vi "Sort Scan Parameters.vi"(8 "error in (no error)":errorcluster, 11 "SweepControl":refnum<class "SMO.SweepControl.lvclass">) -> (0 "error out":errorcluster, 1 "Sorted scan parameters":cluster{T5}[](array[cluster])=[{[{"Start"=0.14, "End"=-0.060000000000000005, "Step"=-0.060000000000000005, "Rate"=0.0, "Waveform type"=enum."linear", "wait (ms or K)"=10000.0, "Address"="Dev2/ao0", "channel"=1}]}, {[{"Start"=0.14, "End"=-0.060000000000000005, "Step"=-0.060000000000000005, "Rate"=0.0, "Waveform type"=enum."linear", "wait (ms or K)"=10000.0, "Address"="Dev2/ao0", "channel"=1}]}, {[{"Start"=0.14, "End"=-0.060000000000000005, "Step"=-0.060000000000000005, "Rate"=0.0, "Waveform type"=enum."linear", "wait (ms or K)"=10000.0, "Address"="Dev2/ao0", "channel"=1}, {"Start"=0.14, "End"=-0.060000000000000005, "Step"=-0.060000000000000005, "Rate"=0.0, "Waveform type"=enum."linear", "wait (ms or K)"=10000.0, "Address"="Dev2/ao0", "channel"=1}]}] {"?"."Rate" format="%.2f"; "?"."Step" format="%#_6p"; "?"."End" format="%#_6p"; "?"."Start" format="%#_6p"}, 2 "Sorted scan control":cluster{T7}[](array[cluster])=[{[{"Priority"=enum."Priority 0", "Scan name"=enum."Delay"}]}, {[{"Priority"=enum."Priority 1", "Scan name"=enum."Lockin Amplitude"}]}, {[{"Priority"=enum."Priority 2", "Scan name"=enum."Lockin Bias"}, {"Priority"=enum."Priority 2", "Scan name"=enum."Magnet Field"}]}], 3 "SweepControl":refnum<class "SMO.SweepControl.lvclass">)   [LabVIEW 2019, in "SMO.SweepControl.lvclass"]
uses:
  SMO.SweepControl.lvclass
  Typedefs/Cluster - ScanParamters.ctl
  Typedefs/ScanParamters.ctl
  Typedefs/Enum - Priority.ctl
  Typedefs/Enum - Action.ctl
  Typedefs/Cluster - ScanControl.ctl
  Typedefs/ScanControl.ctl
  Typedefs/Enum - PostAction - 2.ctl
  Typedefs/Cluster - Sweep Control.ctl
panel:
  out "Sorted scan parameters 2":cluster{"Scan parameters 2":T1[]}[](array[cluster]) {"Scan parameters 2"."Rate" format="%.2f"; "Scan parameters 2"."Step" format="%#_6p"; "Scan parameters 2"."End" format="%#_6p"; "Scan parameters 2"."Start" format="%#_6p"}
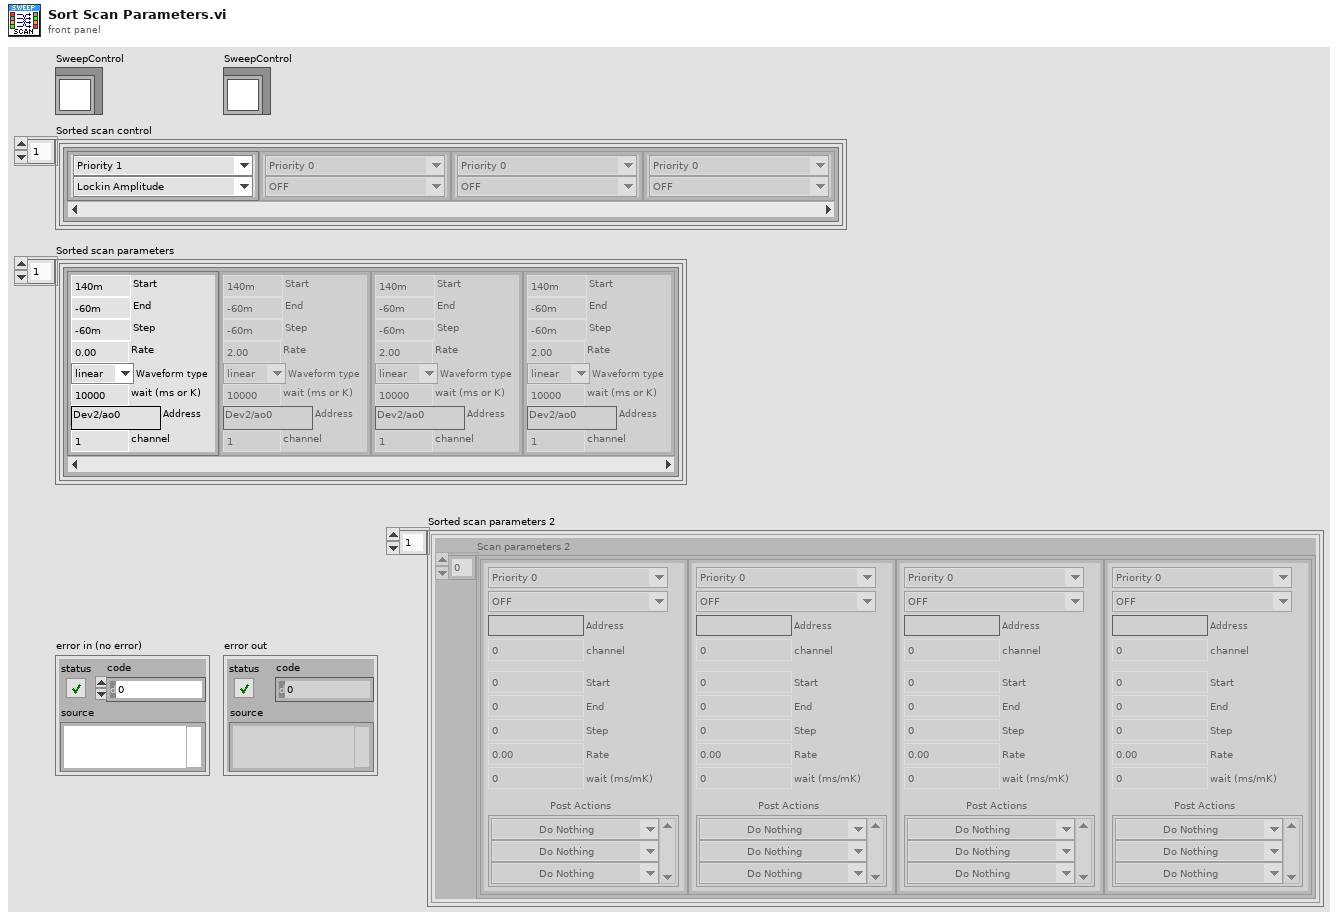
[diagram p1: front panel]
types:
  T1 = typedef "SMO.SweepControl.lvclass/Cluster - Sweep Control.ctl" = cluster{"Start":dbl, "End":dbl, "Step":dbl, "Rate":dbl, "wait (ms/mK)":u32, "Address":string, "Priority":T2, "Scan name":T3, "Post Actions":T4[], "channel":i32}
  T2 = typedef "SMO.SweepControl.lvclass/Enum - Priority.ctl" = enum16{"Priority 0", "Priority 1", "Priority 2", "Priority 3", "Priority 4", "Priority 5"}
  T3 = typedef "SMO.SweepControl.lvclass/Enum - Action.ctl" = enum16{"OFF", "time", "Lockin Amplitude", "Lockin Frequency", "Lockin Bias", "Delay", "Strain", "DAQ Bias", "Magnet Field", "Temperature", "MW f1", "MW f2", "MW Amplitude1", "MW Amplitude2"}
  T4 = typedef "SMO.SweepControl.lvclass/Enum - PostAction - 2.ctl" = enum16{"Do Nothing", "Wait (time)", "Wait (Temperature)", "Wait (<T ; B sweep)", "Wait (Magnet)"}
  T5 = typedef "SMO.SweepControl.lvclass/ScanParamters.ctl" = T6[]
  T6 = typedef "SMO.SweepControl.lvclass/Cluster - ScanParamters.ctl" = cluster{"Start":dbl, "End":dbl, "Step":dbl, "Rate":dbl, "Waveform type":enum16{"linear", "triangle", "power"}, "wait (ms or K)":dbl, "Address":string, "channel":i32}
  T7 = typedef "SMO.SweepControl.lvclass/ScanControl.ctl" = T8[]
  T8 = typedef "SMO.SweepControl.lvclass/Cluster - ScanControl.ctl" = cluster{"Priority":T2, "Scan name":T3}
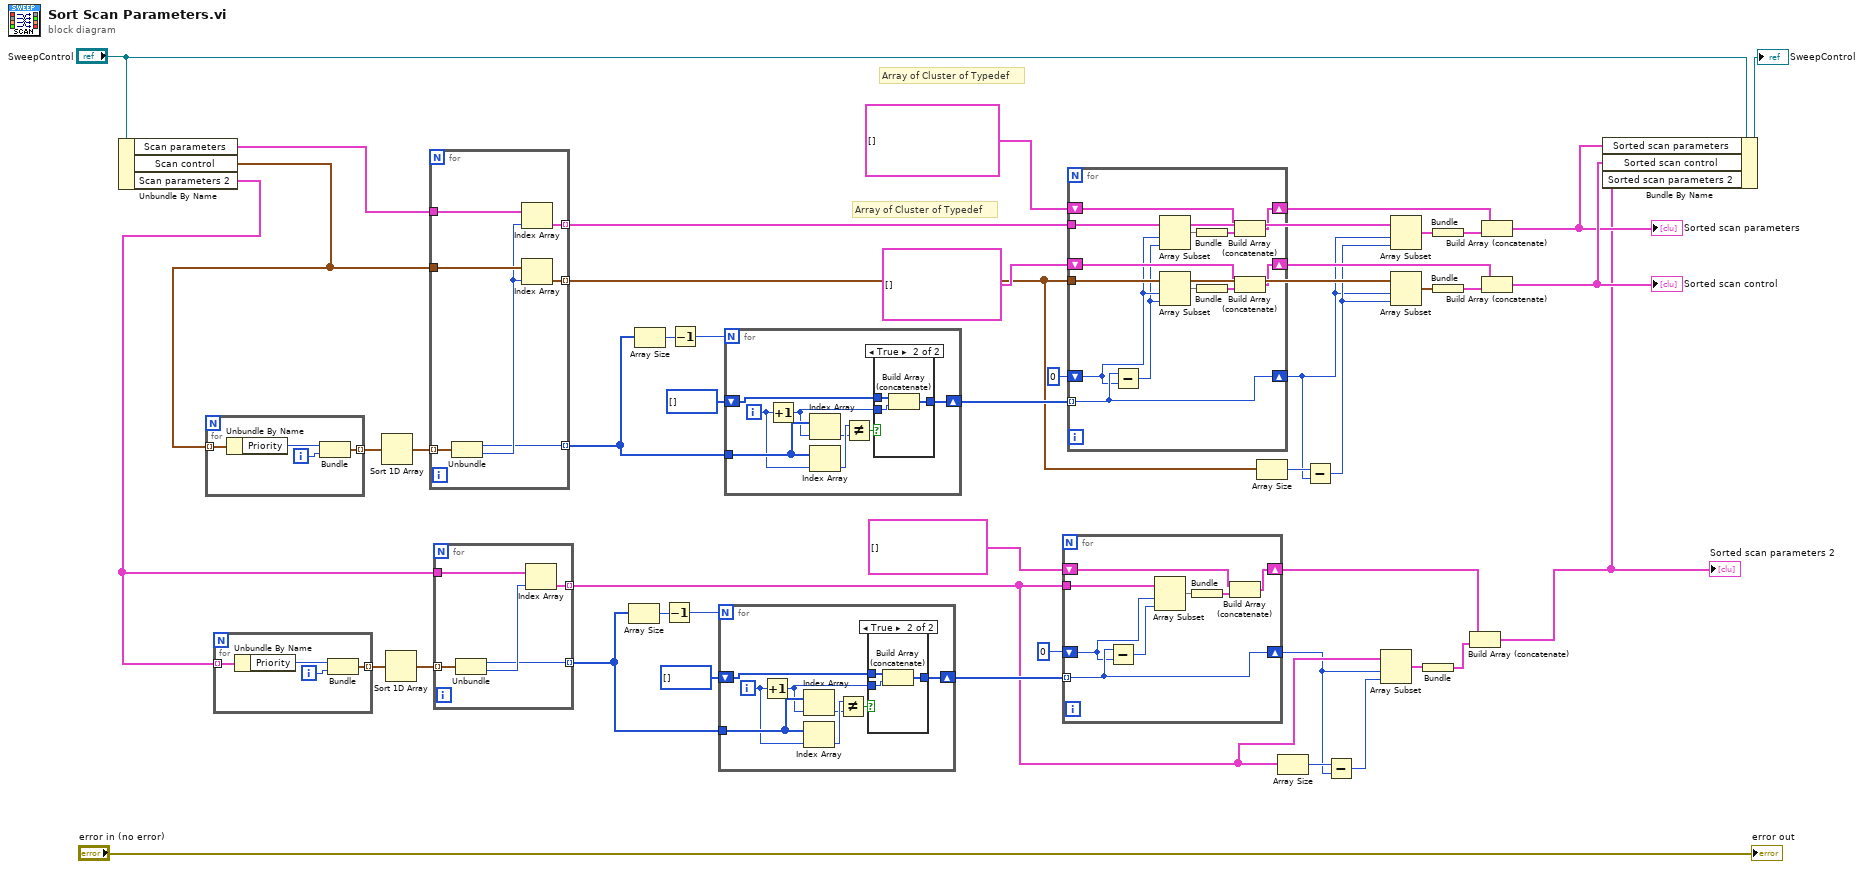
[diagram p0: block diagram]
diagram:
  # "Array of Cluster of Typedef"
  # "Array of Cluster of Typedef"
  n1 = Unbundle By Name("SweepControl") -> ("Scan parameters"=w25:T5, "Scan control"=w20:T7, "Scan parameters 2"=w18:T1[])
  n2 = for {
    tunnel: w20 -> [w47] mode=indexing
    tunnel: [w50] -> w46 mode=indexing
    i -> [w48]
    n3 = Unbundle By Name(w47) -> ("Priority"=w49:T2)
    n4 = Bundle("Priority"=w49, w48) -> (w50:cluster{"Priority":T2, i32})  [unwired: 1 in]
  }
  n5 = for {
    tunnel: w18 -> [w51] mode=indexing
    tunnel: [w54] -> w17 mode=indexing
    i -> [w52]
    n6 = Unbundle By Name(w51) -> ("Priority"=w53:T2)
    n7 = Bundle("Priority"=w53, w52) -> (w54:cluster{"Priority":T2, i32})  [unwired: 1 in]
  }
  n8 = Sort 1D Array(array=w46) -> (sorted array=w45:cluster{"Priority":T2, i32}[])
  n9 = Sort 1D Array(array=w17) -> (sorted array=w16:cluster{"Priority":T2, i32}[])
  n10 = for {
    tunnel: w45 -> [w61] mode=indexing
    tunnel: w20 -> [w60]
    tunnel: [w59] -> w35 mode=indexing
    tunnel: w25 -> [w58]
    tunnel: [w57] -> w31 mode=indexing
    tunnel: [w55] -> w42 mode=indexing
    n11 = Unbundle(w61) -> ("Priority"=w55:T2, w56:i32)
    n12 = Index Array(array=w58, index=w56) -> (element=w57:T6)
    n13 = Index Array(array=w60, index=w56) -> (element=w59:T8)
  }
  n14 = for {
    tunnel: w16 -> [w66] mode=indexing
    tunnel: w18 -> [w65]
    tunnel: [w64] -> w7 mode=indexing
    tunnel: [w62] -> w12 mode=indexing
    n15 = Unbundle(w66) -> ("Priority"=w62:T2, w63:i32)
    n16 = Index Array(array=w65, index=w63) -> (element=w64:T1)
  }
  n17 = Array Size(array=w12) -> (size(s)=w13:i32)
  n18 = Array Size(array=w42) -> (size(s)=w44:i32)
  n19 = Decrement(x=w13) -> (x-1=w14:i32)
  n20 = Decrement(x=w44) -> (x-1=w43:i32)
  n21 = for {
    N: w14 -> [_]
    tunnel: w12 -> [w74]
    shift-right: [w70] -> w10
    shift-left: i32[] [] -> [w69]
    i -> [w67]
    n22 = Increment(x=w67) -> (x+1=w68:i32)
    n23 = Index Array(array=w74, index=w68) -> (element=w71:T2)
    n24 = Index Array(array=w74, index=w67) -> (element=w73:T2)
    n25 = Not Equal?(x=w73, y=w71) -> (x != y?=w72:bool)
    n26 = case shown="True" w72 {
      tunnel: [w75 w78] -> w70
      tunnel: w69 -> [w75 w77]
      tunnel: w68 -> [_ w76]
      frame False {
      }
      frame True {
        n27 = Build Array (concatenate)(w77, w76) -> (w78:i32[])
      }
    }
  }
  n28 = for {
    N: w43 -> [_]
    tunnel: w42 -> [w86]
    shift-right: [w82] -> w39
    shift-left: i32[] [] -> [w81]
    i -> [w79]
    n29 = Increment(x=w79) -> (x+1=w80:i32)
    n30 = Index Array(array=w86, index=w80) -> (element=w83:T2)
    n31 = Index Array(array=w86, index=w79) -> (element=w85:T2)
    n32 = Not Equal?(x=w85, y=w83) -> (x != y?=w84:bool)
    n33 = case shown="True" w84 {
      tunnel: [w87 w90] -> w82
      tunnel: w81 -> [w87 w89]
      tunnel: w80 -> [_ w88]
      frame False {
      }
      frame True {
        n34 = Build Array (concatenate)(w89, w88) -> (w90:i32[])
      }
    }
  }
  n35 = for {
    tunnel: w10 -> [w98] mode=indexing
    shift-right: [w98] -> w3
    shift-left: 0 -> [w96]
    tunnel: w7 -> [w97]
    shift-right: [w93] -> w4
    shift-left: cluster{"Scan parameters 2":T1[]}[] [] -> [w92]
    n36 = Subtract(x=w98, y=w96) -> (x-y=w95:i32)
    n37 = Array Subset(array=w97, index=w96, length=w95) -> (w94:T1[])
    n38 = Bundle(w94) -> (w91:cluster{T1[]})  [unwired: 1 in]
    n39 = Build Array (concatenate)(w92, w91) -> (w93:cluster{"Scan parameters 2":T1[]}[])
  }
  n40 = for {
    tunnel: w39 -> [w106] mode=indexing
    shift-right: [w111] -> w38
    shift-left: cluster{"Scan control":T7}[] [] -> [w110]
    tunnel: w35 -> [w109]
    shift-right: [w106] -> w29
    shift-left: 0 -> [w104]
    tunnel: w31 -> [w105]
    shift-right: [w101] -> w26
    shift-left: cluster{"Scan parameters":T5}[] [] -> [w100]
    n41 = Subtract(x=w106, y=w104) -> (x-y=w103:i32)
    n42 = Array Subset(array=w105, index=w104, length=w103) -> (w102:T6[])
    n43 = Array Subset(array=w109, index=w104, length=w103) -> (w108:T8[])
    n44 = Bundle(w102) -> (w99:cluster{T6[]})  [unwired: 1 in]
    n45 = Bundle(w108) -> (w107:cluster{T8[]})  [unwired: 1 in]
    n46 = Build Array (concatenate)(w100, w99) -> (w101:cluster{"Scan parameters":T5}[])
    n47 = Build Array (concatenate)(w110, w107) -> (w111:cluster{"Scan control":T7}[])
  }
  n48 = Array Size(array=w35) -> (size(s)=w36:i32)
  n49 = Array Size(array=w7) -> (size(s)=w8:i32)
  n50 = Subtract(x=w36, y=w29) -> (x-y=w30:i32)
  n51 = Subtract(x=w8, y=w3) -> (x-y=w2:i32)
  n52 = Array Subset(array=w7, index=w3, length=w2) -> (w6:T1[])
  n53 = Array Subset(array=w31, index=w29, length=w30) -> (w32:T6[])
  n54 = Array Subset(array=w35, index=w29, length=w30) -> (w34:T8[])
  n55 = Bundle(w6) -> (w5:cluster{T1[]})  [unwired: 1 in]
  n56 = Bundle(w32) -> (w28:cluster{T6[]})  [unwired: 1 in]
  n57 = Bundle(w34) -> (w33:cluster{T8[]})  [unwired: 1 in]
  n58 = Build Array (concatenate)(w4, w5) -> (w1:cluster{"Scan parameters 2":T1[]}[])
  "Sorted scan parameters 2" <- w1
  n59 = Build Array (concatenate)(w26, w28) -> (w22:cluster{"Scan parameters":T5}[])
  "Sorted scan parameters" <- w22
  n60 = Build Array (concatenate)(w38, w33) -> (w23:cluster{"Scan control":T7}[])
  "Sorted scan control" <- w23
  n61 = Bundle By Name(cluster="SweepControl", "Sorted scan parameters"=w22, "Sorted scan control"=w23, "Sorted scan parameters 2"=w1) -> (→"SweepControl":refnum<class "SMO.SweepControl.lvclass">)
  "error out" <- "error in (no error)"
